vi "Lester roche prueba corregida.vi"() -> ()   [LabVIEW 2011]
panel:
  out "601-1000 LLenado":bool
  out "301-600 Medio":bool
  out "1-300 Vacio":bool
  out "Tanque":i32(slide) scale=1.0..1000.0
  # "El programa debera de llenar el tanque \nla bomba genera de 1-50 galones, los cuales \nse suman y esta suma se representa por el \ntanque. \nDebera de ir encendiendo los Led de acuerdo \nal volumen de agua del tanque.\ncuando este se llene se detiene el programa \nnota llenando se entiende cuando la suma \nes igual a 1000 o mayor."
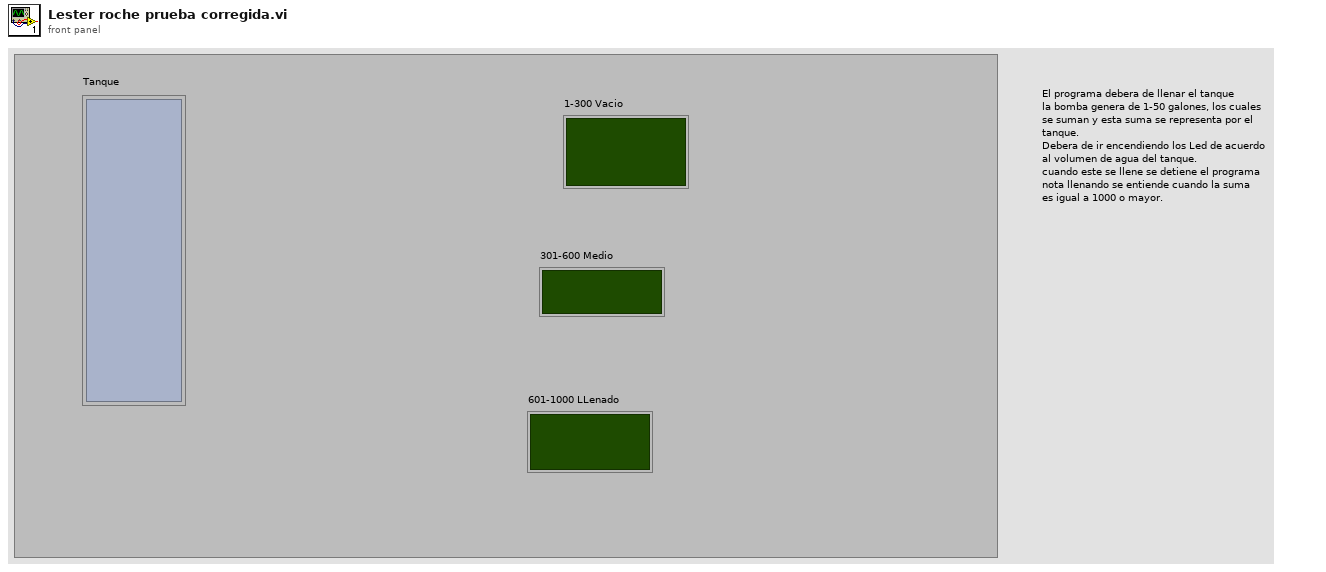
[diagram p1: front panel]
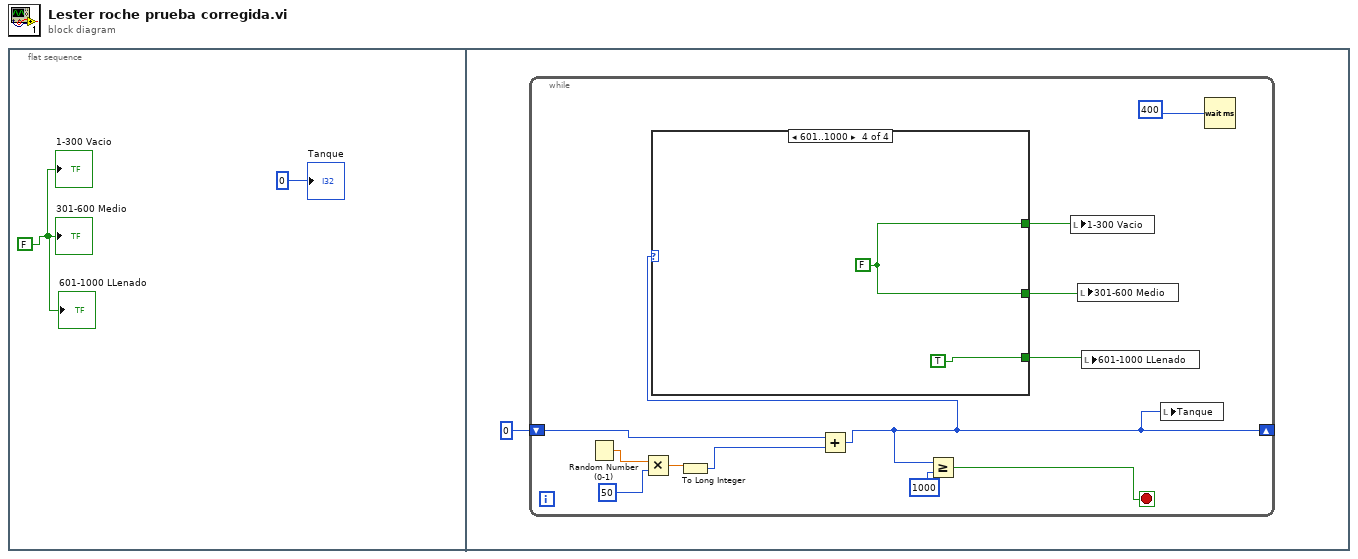
[diagram p0: block diagram]
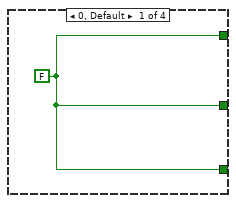
[diagram p2: hidden frame]
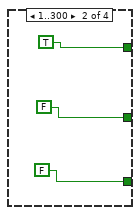
[diagram p3: hidden frame]
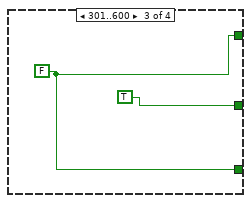
[diagram p4: hidden frame]
diagram:
  n1 = flat-sequence {
    frame #0 {
      w1 = FALSE
      "Tanque" <- 0
      "1-300 Vacio" <- w1
      "301-600 Medio" <- w1
      "601-1000 LLenado" <- w1
    }
    frame #1 {
      n2 = while {
        shift-right: [w5] -> _
        shift-left: 0 -> [w9]
        stop <- w14 stop-if-true
        n3 = Random Number (0-1)() -> (number: 0 to 1=w12:dbl)
        n4 = Multiply(x=w12, y=50) -> (x*y=w13:dbl)
        n5 = To Long Integer(number=w13) -> (32bit integer=w10:i32)
        n6 = Add(x=w9, y=w10) -> (x+y=w5:i32)
        n7 = case shown="601..1000" w5 {
          tunnel: [w16 TRUE w20 w22] -> w8
          tunnel: [w16 FALSE TRUE w22] -> w7
          tunnel: [w16 FALSE w20 TRUE] -> w6
          frame 0, Default {
            w16 = FALSE
          }
          frame 1..300 {
          }
          frame 301..600 {
            w20 = FALSE
          }
          frame 601..1000 {
            w22 = FALSE
          }
        }
        n8 = Greater Or Equal?(x=w5, y=1000) -> (x >= y?=w14:bool)
        n9 = local write "1-300 Vacio"(w8) -> ()
        n10 = local write "301-600 Medio"(w7) -> ()
        n11 = local write "601-1000 LLenado"(w6) -> ()
        n12 = local write "Tanque"(w5) -> ()
        n13 = Wait (ms)(milliseconds to wait=u32 400) -> ()  [unwired: 1 out]
      }
    }
  }
